vi "axis_GetHttpRequest.vi"(6 "Frame Rate":u32(slide) max=30 scale=0.0..30.0, 7 "Compression":u32(slide)=25 scale=0.0..99.0, 11 "Pixel Format":T1(ring)=enum."320 x 240 MJPG") -> (3 "HTTP Request":string)   [LabVIEW 2012]
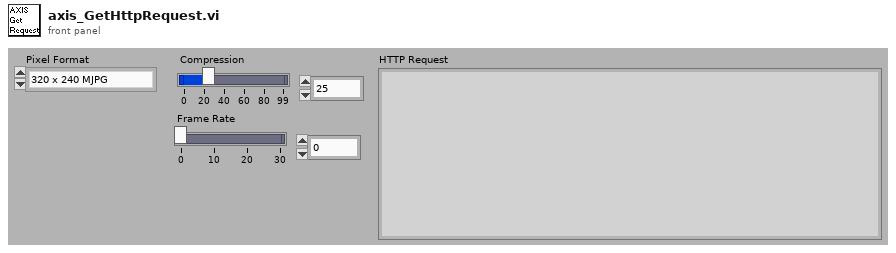
[diagram p1: front panel]
types:
  T1 = enum16{"640 x 480 MJPG", "320 x 240 MJPG", "160 x 120 MJPG"}
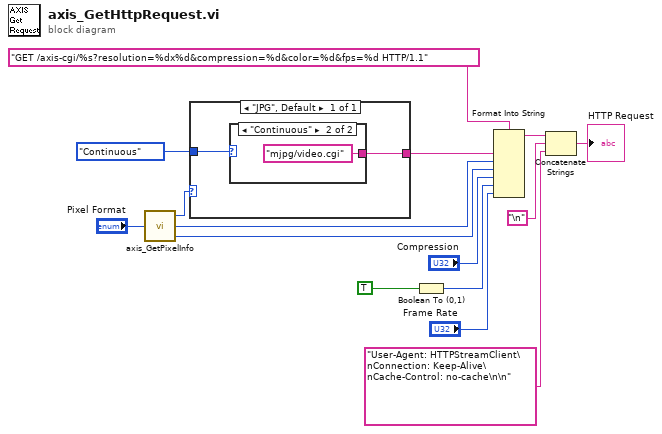
[diagram p0: block diagram]
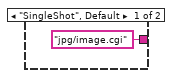
[diagram p2: hidden frame]
diagram:
  n1 = call "axis_GetPixelInfo.vi"("Pixel Format"="Pixel Format") -> ("Type"=w6:enum16{"JPG"}, "Width"=w14:u32, "Height"=w15:u32)
  n2 = case shown="\"JPG\", Default" w6 {
    tunnel: [w17] -> w2
    tunnel: enum16{"SingleShot", "Continuous"}."Continuous" ("Acquisition Type") -> [w16]
    frame "JPG", Default {
      n3 = case shown="\"Continuous\"" w16 {
        tunnel: ["jpg/image.cgi" "mjpg/video.cgi"] -> w17
        frame "SingleShot", Default {
        }
        frame "Continuous" {
        }
      }
    }
  }
  n4 = Boolean To (0,1)(Boolean=TRUE ("Color?")) -> (0, 1=w3:i16)
  n5 = Format Into String(format string="GET /axis-cgi/%s?resolution=%dx%d&compression=%d&color=%d&fps=%d HTTP/1.1", w2, w14, w15, "Compression", w3, "Frame Rate") -> (resulting string=w8:string)  [unwired: 2 in, 1 out]
  n6 = Concatenate Strings(w8, "\n", "User-Agent: HTTPStreamClient\nConnection: Keep-Alive\nCache-Control: no-cache\n\n") -> (→"HTTP Request":string)
